vi "Galil_arrayDownload.vi"() -> ()   [LabVIEW 2011]
panel:
  in  "Galil.IGalil":refnum<k7>
  out "Library Version:":string
  out "Array Name":string
  out "Uploaded Array:":dbl[](array[numeric])
  out "error out":errorcluster
  out "Connected To:":string
  in  "Connection String:":string
  # "This vi Shows how to use the arrayDownload function of the Galil Communications Library.  \n\nIf Connection String is left blank, the vi will open the connections dialog when run.  If a value is input into Connection String, the vi will attempt to connect to the controller at that address (ex COM1 19200).\n\nThe vi uses an Array Constant for the arrayDownload function to download the array to the controller.  It then uploads the array from the controller with the arrayUpload function and shows it on the front Panel"
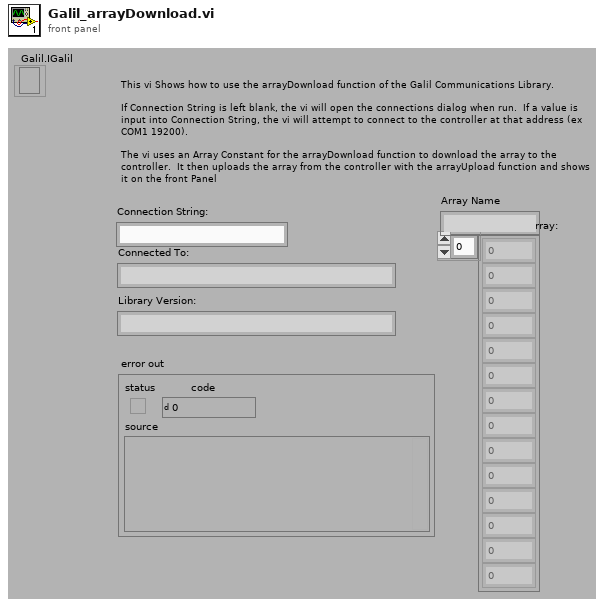
[diagram p1: front panel]
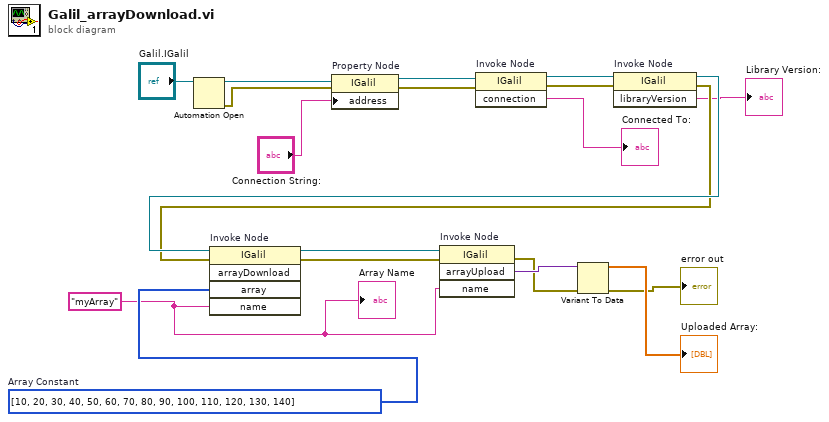
[diagram p0: block diagram]
diagram:
  w11 = "myArray"
  w14 = i32[] [10, 20, 30, 40, 50, 60, 70, 80, 90, 100, 110, 120, 130, 140]  # Array Constant
  n1 = Automation Open(Automation Refnum="Galil.IGalil") -> (Automation Refnum=w20:refnum<k7>, error out=w18:errorcluster)  [unwired: 1 in, 2 out]
  n2 = property on="Property Node" class="IGalil"(reference=w20, error in=w18, "address"="Connection String:") -> (reference out=w19:refnum<k7>, error out=w17:errorcluster)
  n3 = invoke on="Invoke Node" class="IGalil" method="connection"(reference=w19, error in=w17) -> (reference out=w6:refnum<k7>, error out=w4:errorcluster, "connection"=→"Connected To:":string)  [unwired: 1 in]
  n4 = invoke on="Invoke Node" class="IGalil" method="libraryVersion"(reference=w6, error in=w4) -> (reference out=w5:refnum<k7>, error out=w3:errorcluster, "libraryVersion"=→"Library Version:":string)  [unwired: 1 in]
  n5 = invoke on="Invoke Node" class="IGalil" method="arrayDownload"(reference=w5, error in=w3, "array"=w14, "name"=w11) -> (reference out=w13:refnum<k7>, error out=w12:errorcluster)  [unwired: 1 in, 3 out]
  n6 = invoke on="Invoke Node" class="IGalil" method="arrayUpload"(reference=w13, error in=w12, "name"=w11) -> (error out=w9:errorcluster, "arrayUpload"=w10:variant)  [unwired: 1 in, 2 out]
  n7 = Variant To Data(error in=w9, Variant=w10) -> (data=→"Uploaded Array:":dbl[], error out=→"error out":errorcluster)  [unwired: 1 in]
  "Array Name" <- w11
